vi "Write Both Fan States.vi"(8 "error in (no error)":cluster{"状态":bool, "代码":i32, "源":string} caption="错误输入（无错误）", 9 "风扇B状态":bool, 10 "风扇A状态":bool, 11 "双风扇输入":refnum<class "Dual Fan.lvclass">) -> (0 "error out":cluster{"状态":bool, "代码":i32, "源":string} caption="错误输出")   [LabVIEW 2015, in "Dual Fan.lvlib" / "Dual Fan.lvclass"]
doc: "子类中必须对该方法进行重写以设置风扇状态。“真”表示打开风扇，“假”表示关闭风扇。不能保证该方法仅用于状态转移－风扇已处于指定状态下时也可能调用该方法。"
uses:
  Dual Fan.lvclass
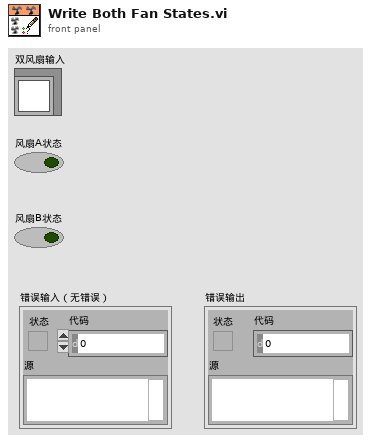
[diagram p1: front panel]
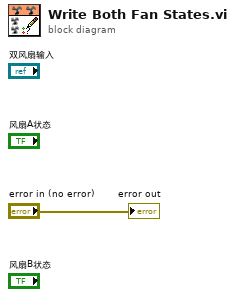
[diagram p0: block diagram]
diagram:
  "error out" <- "error in (no error)"
